vi "HatchPanel.vi"   [LabVIEW 2018]
uses:
  hatchPanelEnum.ctl
  <vilib>/Platform/TimedLoop/XDataNode/timing_clust.ctl
  <vilib>/Platform/TimedLoop/XDataNode/nitl_modes.ctl
  <vilib>/Platform/TimedLoop/XDataNode/wakeup.ctl
  <vilib>/Rock Robotics/WPI/Solenoid/WPI_SolenoidValue.ctl
  <vilib>/Rock Robotics/WPI/Solenoid/WPI_SolenoidSetEnum.vi
  <vilib>/platform/TimedLoop/XDataNode/XDataNode.xnode
  <vilib>/Platform/TimedLoop/XDataNode/XDNodeRunTimeDep.lvlib
types:
  T1 = typedef "hatchPanelEnum.ctl" = enum16{"Stop", "Forward", "Backward"}
  T2 = typedef "XDNodeRunTimeDep.lvlib/timing_clust.ctl" = cluster{"Expected End [f-1]":u64, "Actual End [f-1]":u64, "Finished Late? [f-1]":bool, "Expected End [i-1]":u64, "Actual End [i-1]":u64, "Finished Late? [i-1]":bool, "Expected Start [i]":u64, "Actual Start [i]":u64, "Expected Start [f]":u64, "Actual Start [f]":u64, "Source Name":string, "Structure Name":string, "Period":i64, "Deadline":i64, "Offset":i64, "Start":i64, "Priority":i32, "Timeout":i32, "Mode":T3, "Wakeup Reason":T4, "Error":errorcluster, "Source Type":string, "Secondary Source Type":string, "Global End Time":u64, "Global Start Time":u64, "Frame Duration":u64, "Iteration Duration":u64, "Assigned CPU":i32, "I/O Scan Engine Mode":u32}
  T3 = typedef "XDNodeRunTimeDep.lvlib/nitl_modes.ctl" = enum32{"No Change", "Process missed periods, maintain original phase", "Discard missed periods, maintain original phase", "Process missed periods, ignore original phase", "Discard missed periods, ignore original phase"}
  T4 = typedef "XDNodeRunTimeDep.lvlib/wakeup.ctl" = enum32{"Normal", "Aborted", "Asynchronous wakeup", "Timing source error", "Timed loop error", "Timeout"}
  T5 = typedef "WPI_SolenoidDevRef.ctl" = cluster{"DevStatus":errorcluster, "Pneumatics Control Module":u8, "Forward Solenoid Channel":T6, "Reverse Solenoid Channel":T6}
  T6 = typedef "WPI_SolenoidChannel.ctl" = enum8{"Solenoid 0", "Solenoid 1", "Solenoid 2", "Solenoid 3", "Solenoid 4", "Solenoid 5", "Solenoid 6", "Solenoid 7", "Invalid"}
  T7 = typedef "WPI_SolenoidValue.ctl" = enum16{"Off", "On", "Forward", "Reverse"}
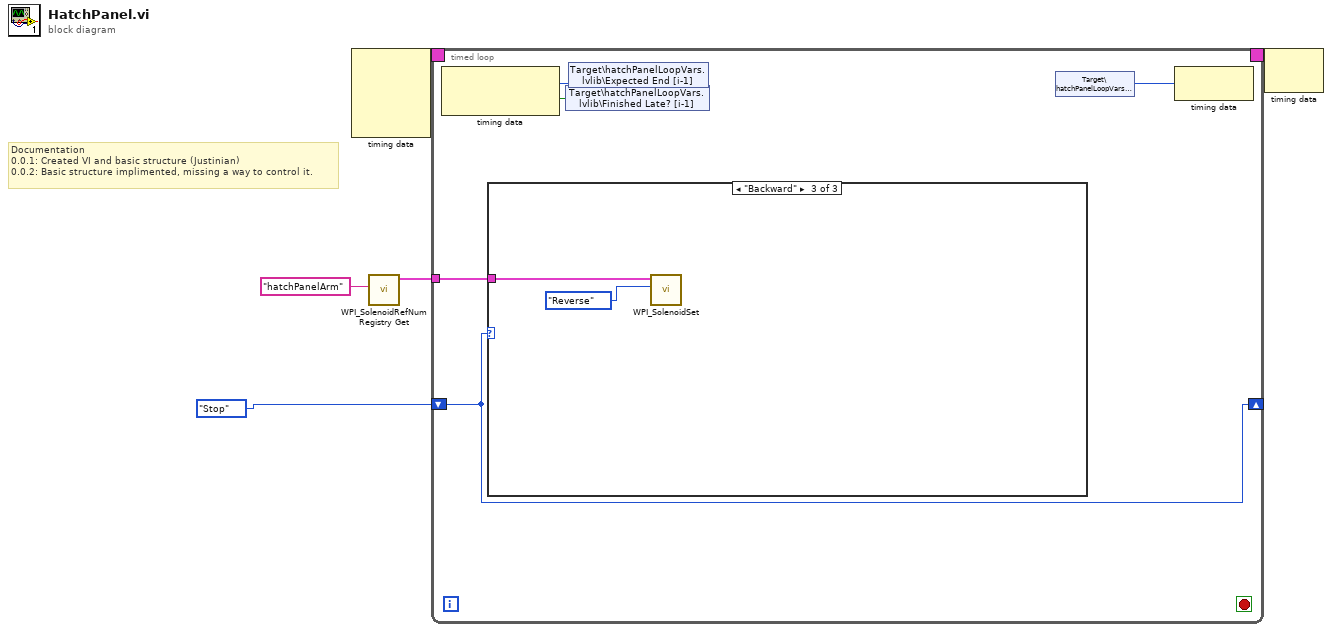
[diagram p0: block diagram]
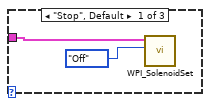
[diagram p2: hidden frame]
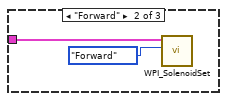
[diagram p3: hidden frame]
diagram:
  # "Documentation\n0.0.1: Created VI and basic structure (Justinian)\n0.0.2: Basic structure implimented, missing a way to control it."
  n1 = node-c288() -> (w5:T2)  [unwired: 4 in]
  n2 = call <vilib>:"WPI_SolenoidRefNum Registry Get.vi"("refnum name"="hatchPanelArm") -> ("SolenoidDevRef"=w2:T5)  [unwired: 9 in, 1 out]
  n3 = timed-loop {
    timing: w5 -> [_]
    timing-out: [_] -> w4
    shift-right: [w6] -> _
    shift-left: hatchPanelEnum."Stop" -> [w6]
    tunnel: w2 -> [w10]
    stop <- _ stop-if-true
    n4 = node-c288() -> (w9:i64, w8:bool)  [unwired: 1 in]
    n5 = case shown="\"Backward\"" w6 {
      tunnel: w10 -> [w12 w14 w16]
      frame "Stop", Default {
        n6 = call-poly <vilib>:"WPI_SolenoidSet.vi"("Value"=WPI_SolenoidValue."Off", "SolenoidDevRef"=w12) -> ()  [unwired: 8 in, 2 out]
      }
      frame "Forward" {
        n7 = call-poly <vilib>:"WPI_SolenoidSet.vi"("Value"=WPI_SolenoidValue."Forward", "SolenoidDevRef"=w14) -> ()  [unwired: 8 in, 2 out]
      }
      frame "Backward" {
        n8 = call-poly <vilib>:"WPI_SolenoidSet.vi"("Value"=WPI_SolenoidValue."Reverse", "SolenoidDevRef"=w16) -> ()  [unwired: 8 in, 2 out]
      }
    }
    n9 = shared-variable "Target\\hatchPanelLoopVars.lvlib\\Finished Late? [i-1]"(w8) -> ()  [unwired: 1 in, 1 out]
    n10 = shared-variable "Target\\hatchPanelLoopVars.lvlib\\Expected End [i-1]"(w9) -> ()  [unwired: 1 in, 1 out]
    n11 = shared-variable "Target\\hatchPanelLoopVars.lvlib\\Period"() -> (w7:i64)  [unwired: 1 in, 1 out]
    n12 = node-c288(w7) -> ()  [unwired: 1 out]
  }
  n13 = node-c288(w4) -> ()  [unwired: 1 out]
